vi "slink set trigger.vi"(5 "ChannelEnable":cluster{"Channel 1":T1, "Channel 2":T1}, 6 "Numeric":i32, 7 "Channel 1":T1, 8 "error in (no error)":errorcluster, 9 "Simulation":T1, 10 "Command":string, 11 "VISA Refnum in":refnum<visa-resource-name>) -> (0 "error out":errorcluster, 3 "VISA Refnum out":refnum<visa-resource-name>)   [LabVIEW 2020, in "Gentec Slink.lvclass"]
uses:
  Gentec Slink.lvclass
  shared/OnOffTypeDef.ctl
  Serial Commands Slink.ctl
  shared/CompressAndUpdate(Poly)/CompressAndUpdate(Enum).vi
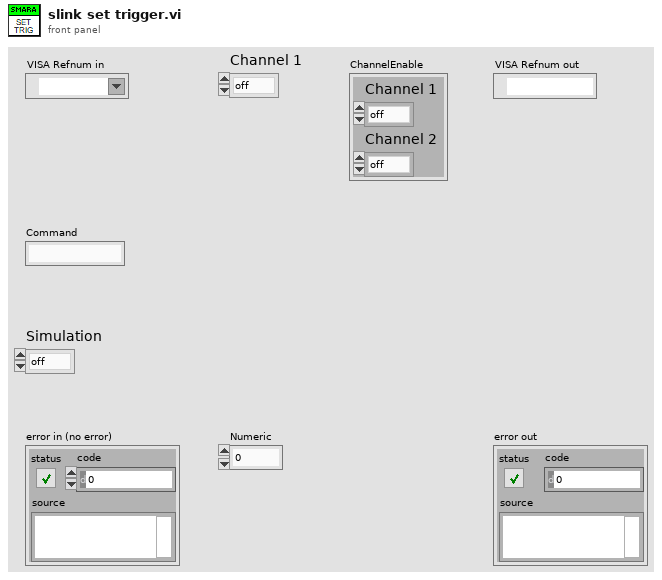
[diagram p1: front panel]
types:
  T1 = typedef "OnOffTypeDef.ctl" = enum16{"off", "on"}
  T2 = typedef "Serial Commands Slink.ctl" = i32
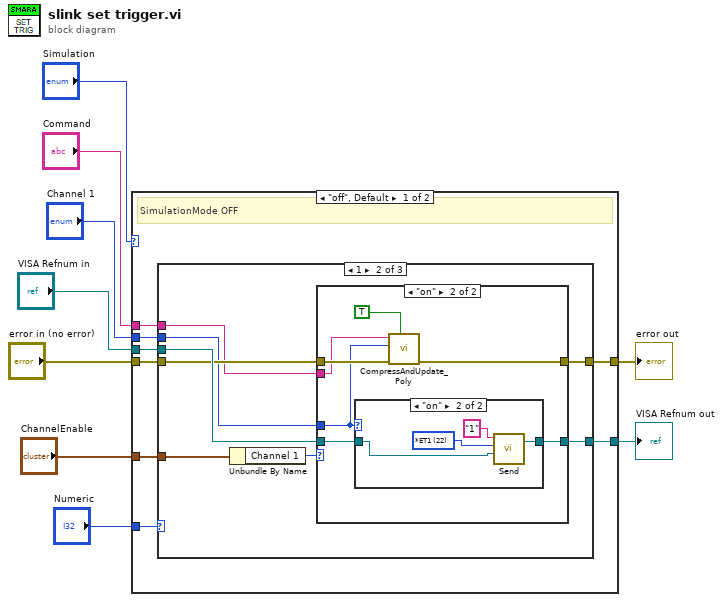
[diagram p0: block diagram]
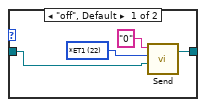
[diagram p4: hidden frame]
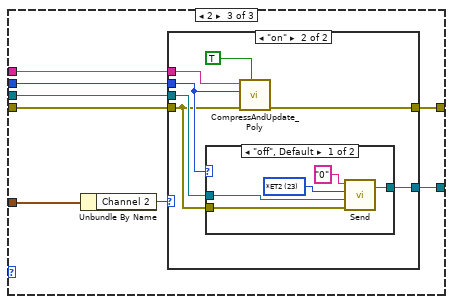
[diagram p5: hidden frame]
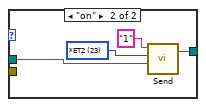
[diagram p7: hidden frame]
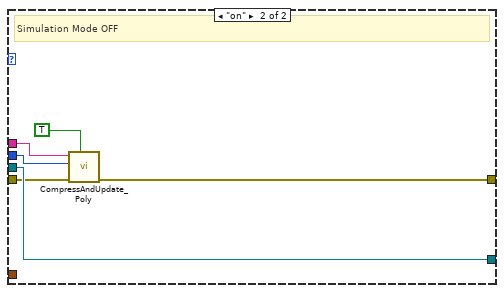
[diagram p8: hidden frame]
diagram:
  n1 = case shown="\"off\", Default" "Simulation" {
    tunnel: "Numeric" -> [w17 _]
    tunnel: [w10 w76] -> w2
    tunnel: "VISA Refnum in" -> [w16 w76]
    tunnel: "Channel 1" -> [w15 w71]
    tunnel: "error in (no error)" -> [w14 w74]
    tunnel: [w13 w73] -> w6
    tunnel: "Command" -> [w12 w72]
    tunnel: "ChannelEnable" -> [w11 _]
    frame "off", Default {
      # "SimulationMode OFF"
      n2 = case shown="1" w17 {
        tunnel: w16 -> [w19 w27 w52]
        tunnel: [w19 w26 w51] -> w10
        tunnel: w15 -> [_ w23 w48]
        tunnel: w14 -> [w18 w25 w50]
        tunnel: [w18 w24 w49] -> w13
        tunnel: w12 -> [_ w22 w47]
        tunnel: w11 -> [_ w21 w46]
        frame 0, Default {
        }
        frame 1 {
          n3 = Unbundle By Name(w21) -> ("Channel 1"=w20:T1)
          n4 = case shown="\"on\"" w20 {
            tunnel: w27 -> [w29 w36]
            tunnel: [w29 w35] -> w26
            tunnel: w25 -> [w28 w33]
            tunnel: [w28 w32] -> w24
            tunnel: w23 -> [_ w31]
            tunnel: w22 -> [_ w30]
            frame "off", Default {
            }
            frame "on" {
              n5 = case shown="\"on\"" w31 {
                tunnel: w36 -> [w38 w42]
                tunnel: [w37 w41] -> w35
                frame "off", Default {
                  w39 = T2 22 items=["*RST", "*VER", "*CA1", "*CA2", "*SS1", "*SS2", "*SU1", "*SU2", "*SD1", "*SD2", "*CS1", "*CS2", "*AT1", "*AT2", "*AN1", "*AN2", "*PW1", "*PW2", "*TL1", "*TL2", "*ST1", "*ST2", "*ET1", "*ET2", "*EM1", "*EM2", "*SC1", "*SC2"] ("string to write")
                  n6 = call "Send.vi"("port number"=w38, "string to write"=w39, "Option"="0") -> ("port out"=w37:refnum<visa-resource-name>)  [unwired: 1 in, 1 out]
                }
                frame "on" {
                  w43 = T2 22 items=["*RST", "*VER", "*CA1", "*CA2", "*SS1", "*SS2", "*SU1", "*SU2", "*SD1", "*SD2", "*CS1", "*CS2", "*AT1", "*AT2", "*AN1", "*AN2", "*PW1", "*PW2", "*TL1", "*TL2", "*ST1", "*ST2", "*ET1", "*ET2", "*EM1", "*EM2", "*SC1", "*SC2"] ("string to write")
                  n7 = call "Send.vi"("port number"=w42, "string to write"=w43, "Option"="1") -> ("port out"=w41:refnum<visa-resource-name>)  [unwired: 1 in, 1 out]
                }
              }
              n8 = call-poly "CompressAndUpdate_Poly.vi"("force CVT update (false)"=TRUE, "error in"=w33, "enum variant"=w31, "command or variable name"=w30) -> ("error out"=w32:errorcluster)  [unwired: 7 in]
            }
          }
        }
        frame 2 {
          n9 = Unbundle By Name(w46) -> ("Channel 2"=w45:T1)
          n10 = case shown="\"on\"" w45 {
            tunnel: w52 -> [w54 w61]
            tunnel: [w54 w60] -> w51
            tunnel: w50 -> [w53 w55]
            tunnel: [w53 w58] -> w49
            tunnel: w48 -> [_ w57]
            tunnel: w47 -> [_ w56]
            frame "off", Default {
            }
            frame "on" {
              n11 = case shown="\"off\", Default" w57 {
                tunnel: w61 -> [w64 w68]
                tunnel: [w63 w67] -> w60
                tunnel: w55 -> [w62 _]
                frame "off", Default {
                  w65 = T2 23 items=["*RST", "*VER", "*CA1", "*CA2", "*SS1", "*SS2", "*SU1", "*SU2", "*SD1", "*SD2", "*CS1", "*CS2", "*AT1", "*AT2", "*AN1", "*AN2", "*PW1", "*PW2", "*TL1", "*TL2", "*ST1", "*ST2", "*ET1", "*ET2", "*EM1", "*EM2", "*SC1", "*SC2"] ("string to write")
                  n12 = call "Send.vi"("error in (no error)"=w62, "port number"=w64, "string to write"=w65, "Option"="0") -> ("port out"=w63:refnum<visa-resource-name>)  [unwired: 1 out]
                }
                frame "on" {
                  w69 = T2 23 items=["*RST", "*VER", "*CA1", "*CA2", "*SS1", "*SS2", "*SU1", "*SU2", "*SD1", "*SD2", "*CS1", "*CS2", "*AT1", "*AT2", "*AN1", "*AN2", "*PW1", "*PW2", "*TL1", "*TL2", "*ST1", "*ST2", "*ET1", "*ET2", "*EM1", "*EM2", "*SC1", "*SC2"] ("string to write")
                  n13 = call "Send.vi"("port number"=w68, "string to write"=w69, "Option"="1") -> ("port out"=w67:refnum<visa-resource-name>)  [unwired: 1 in, 1 out]
                }
              }
              n14 = call-poly "CompressAndUpdate_Poly.vi"("force CVT update (false)"=TRUE, "error in"=w55, "enum variant"=w57, "command or variable name"=w56) -> ("error out"=w58:errorcluster)  [unwired: 7 in]
            }
          }
        }
      }
    }
    frame "on" {
      # "Simulation Mode OFF"
      n15 = call-poly "CompressAndUpdate_Poly.vi"("force CVT update (false)"=TRUE, "error in"=w74, "enum variant"=w71, "command or variable name"=w72) -> ("error out"=w73:errorcluster)  [unwired: 7 in]
    }
  }
  "error out" <- w6
  "VISA Refnum out" <- w2
